vi "Gunsim Simulate.vi"(1 "Robot Constants":T4={"Distance from Pivot Point to Drive Mount(in)"=2.0, "Distance from Pivot Point to Arm Mount(in)"=2.0, "Distance from Pivot Point to Launcher(in)"=2.0, "Distance from Pivot Point to Camera(in)"=2.0, "WheelEncoder Ticks/Revolution"=2.0, "Wheel Radius"=2.0, "Triangle Angle(degrees)"=2.0, "Minimum LA Distance(inches)"=2.0, "LA Distance/Tick(inches)"=2.0}, 2 "cluster in":T3, 3 "Other Constants":T2={"Ball Diameter(in)"=10.0, "Air Density(g/in^3)"=0.02, "Drag coefficient"=0.5, "Ball Mass(g)"=300.0, "gravity(in/s^2)"=-386.09, "Minimum Goal Height(in)"=90.0, "Maximum Goal Height(in)"=104.0}, 4 "Parameters":T1) -> (0 "Range":T5)   [LabVIEW 2015]
panel:
  out "XY Graph":cluster{dbl[], dbl[]}(graph)
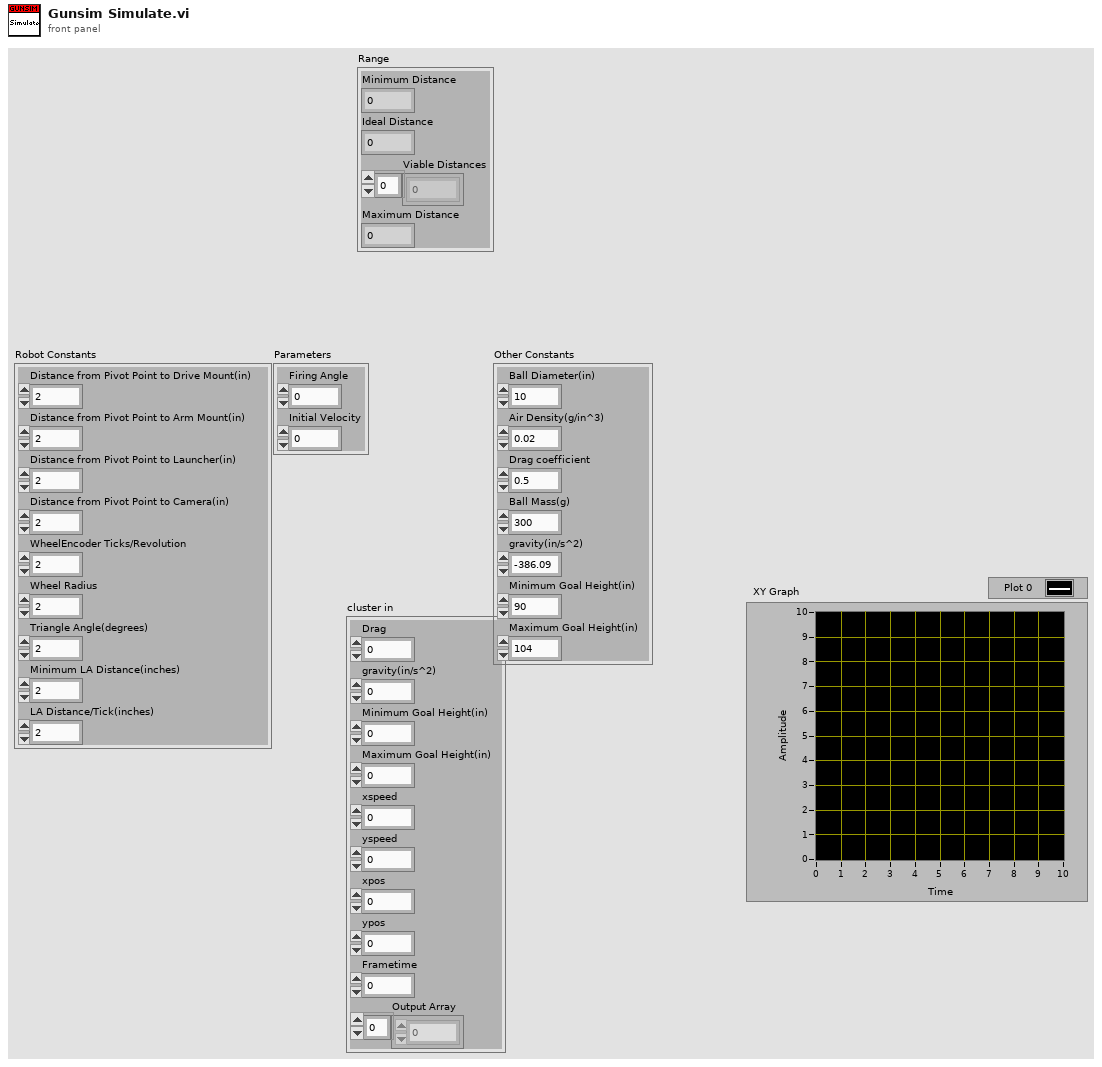
[diagram p1: front panel]
types:
  T1 = cluster{"Firing Angle":dbl, "Initial Velocity":dbl}
  T2 = cluster{"Ball Diameter(in)":dbl, "Air Density(g/in^3)":dbl, "Drag coefficient":dbl, "Ball Mass(g)":dbl, "gravity(in/s^2)":dbl, "Minimum Goal Height(in)":dbl, "Maximum Goal Height(in)":dbl}
  T3 = cluster{"Drag":dbl, "gravity(in/s^2)":dbl, "Minimum Goal Height(in)":dbl, "Maximum Goal Height(in)":dbl, "xspeed":dbl, "yspeed":dbl, "xpos":dbl, "ypos":dbl, "Frametime":dbl, "Output Array":dbl[]}
  T4 = cluster{"Distance from Pivot Point to Drive Mount(in)":dbl, "Distance from Pivot Point to Arm Mount(in)":dbl, "Distance from Pivot Point to Launcher(in)":dbl, "Distance from Pivot Point to Camera(in)":dbl, "WheelEncoder Ticks/Revolution":dbl, "Wheel Radius":dbl, "Triangle Angle(degrees)":dbl, "Minimum LA Distance(inches)":dbl, "LA Distance/Tick(inches)":dbl}
  T5 = cluster{"Minimum Distance":dbl, "Ideal Distance":dbl, "Viable Distances":dbl[], "Maximum Distance":dbl}
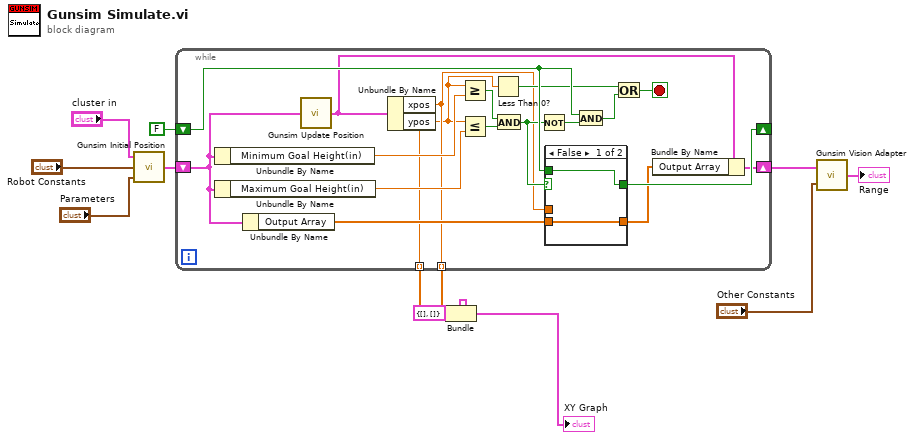
[diagram p0: block diagram]
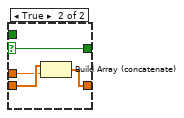
[diagram p2: hidden frame]
diagram:
  n1 = call "Gunsim Initial Position.vi"("Parameters"="Parameters", "Robot Constants"="Robot Constants", "cluster in"="cluster in") -> ("cluster out"=w9:T3)
  n2 = while {
    shift-right: [w25] -> _
    shift-left: FALSE -> [w24]
    shift-right: [w15] -> w10
    shift-left: w9 -> [w19]
    tunnel: [w14] -> w4 mode=indexing
    tunnel: [w13] -> w3 mode=indexing
    stop <- w20 stop-if-true
    n3 = Unbundle By Name(w19) -> ("Minimum Goal Height(in)"=w27:dbl)
    n4 = Unbundle By Name(w19) -> ("Maximum Goal Height(in)"=w28:dbl)
    n5 = Unbundle By Name(w19) -> ("Output Array"=w18:dbl[])
    n6 = call "Gunsim Update Position.vi"("cluster in"=w19) -> ("cluster out"=w17:T3)
    n7 = Unbundle By Name(w17) -> ("xpos"=w14:dbl, "ypos"=w13:dbl)
    n8 = Greater Or Equal?(x=w13, y=w27) -> (x >= y?=w30:bool)
    n9 = Less Or Equal?(x=w13, y=w28) -> (x <= y?=w29:bool)
    n10 = Less Than 0?(x=w13) -> (x < 0?=w22:bool)
    n11 = And(x=w30, y=w29) -> (x .and. y?=w23:bool)
    n12 = Not(x=w23) -> (.not. x?=w26:bool)
    n13 = case shown="False" w23 {
      selector: w23 -> [_ w36]
      tunnel: w14 -> [_ w34]
      tunnel: w18 -> [w32 w35]
      tunnel: [w32 w33] -> w16
      tunnel: [w31 w36] -> w25
      tunnel: w24 -> [w31 _]
      frame False {
      }
      frame True {
        n14 = Build Array (concatenate)(w35, w34) -> (w33:dbl[])
      }
    }
    n15 = And(x=w24, y=w26) -> (x .and. y?=w21:bool)
    n16 = Or(x=w22, y=w21) -> (x .or. y?=w20:bool)
    n17 = Bundle By Name(cluster=w17, "Output Array"=w16) -> (w15:T3)
  }
  n18 = Bundle(cluster=cluster{dbl[], dbl[]} {[], []}, w4, w3) -> (→"XY Graph":cluster{dbl[], dbl[]})
  n19 = call "Gunsim Vision Adapter.vi"("Other Constants"="Other Constants", "cluster in"=w10) -> ("cluster out"=→"Range":T5)
